vi "Get SMO Public API.vi"(8 "error in (no error)":errorcluster, 11 "Inst.RP100 in":refnum<class "Inst.RP100.lvclass">) -> (0 "error out":errorcluster, 2 "Commands":string[](array[string]), 3 "Inst.RP100 out":refnum<class "Inst.RP100.lvclass">)   [LabVIEW 2019, in "Inst.RP100.lvlib" / "Inst.RP100.lvclass"]
uses:
  Inst.RP100.lvclass
  <userlib>/LevyLab/Instrument Framework/Instrument Types/Strain/Instrument.Strain.lvclass
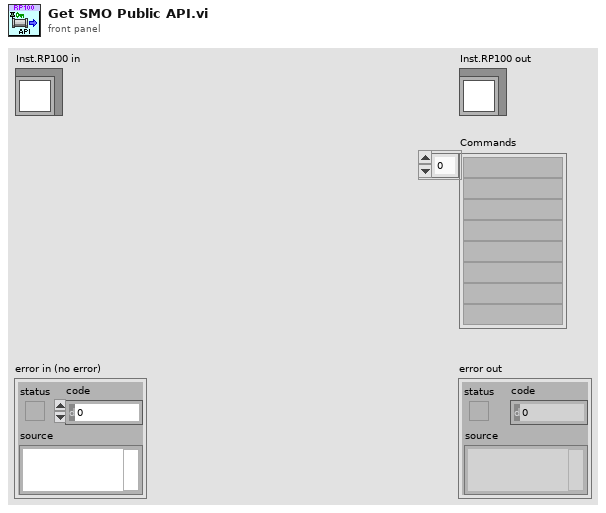
[diagram p1: front panel]
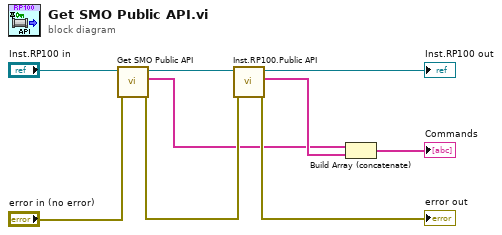
[diagram p0: block diagram]
diagram:
  n1 = call-parent "Get SMO Public API.vi"("error in (no error)"="error in (no error)", "Instrument.Strain in"="Inst.RP100 in") -> ("error out"=w4:errorcluster, "commands"=w2:string[], "Instrument.Strain out"=w1:refnum<class "Inst.RP100.lvclass">)  [unwired: 7 in]
  n2 = call "Inst.RP100.Public API.vi"("error in (no error)"=w4, "Inst.RP100 in"=w1) -> ("error out"=→"error out":errorcluster, "commands (this level)"=w3:string[], "Inst.RP100 out"=→"Inst.RP100 out":refnum<class "Inst.RP100.lvclass">)  [unwired: 7 in]
  n3 = Build Array (concatenate)(w2, w3) -> (→"Commands":string[])
